vi "Read ROI Name.vi"(8 "error in (no error)":errorcluster, 11 "Select Report File Dialog in":refnum<class "ROI Name Dialog.lvclass">) -> (0 "error out":errorcluster, 2 "Select Report File":string, 3 "Select Report File Dialog out":refnum<class "ROI Name Dialog.lvclass">)   [LabVIEW 2014, in "ROI Name Dialog.lvlib" / "ROI Name Dialog.lvclass"]
uses:
  ROI Name Dialog.lvclass
  ROI Name Dialog.lvclass/ROI Name Dialog.ctl
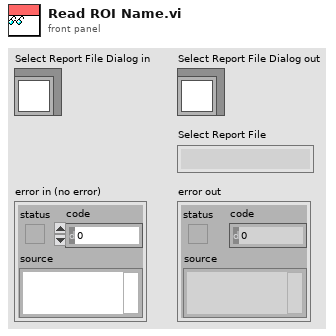
[diagram p1: front panel]
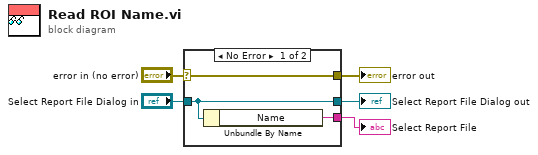
[diagram p0: block diagram]
diagram:
  n1 = case shown="No Error" "error in (no error)" {
    selector: "error in (no error)" -> [w8 w9]
    tunnel: [w8 w9] -> w4
    tunnel: [w7 w10] -> w2
    tunnel: "Select Report File Dialog in" -> [w7 w10]
    tunnel: [w6 _] -> w1
    frame No Error {
      n2 = Unbundle By Name(w7) -> ("Name"=w6:string)
    }
    frame Error {
    }
  }
  "error out" <- w4
  "Select Report File Dialog out" <- w2
  "Select Report File" <- w1
